vi "appendXMLDetectParam.vi"(8 "Detection Parameters":T1, 9 "error in (no error)":errorcluster, 10 "Parent Device Node":refnum<k20>, 11 "DOM document in":refnum<k20>) -> (0 "error out":errorcluster)   [LabVIEW 2013]
uses:
  <resource>/objmgr/DOMUserDefRef.rc
panel:
  out "R%":sgl
  out "Ry":i32
  out "Rx":i32
  out "Max Intensity%":u8
  out "Max Intensity":i32
  out "Treshold":u8
  out "Contrast":i32
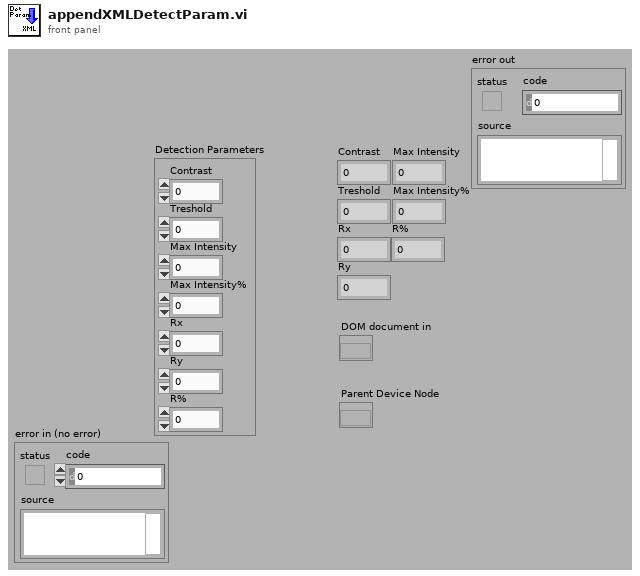
[diagram p1: front panel]
types:
  T1 = cluster{"Contrast":i32, "Treshold":u8, "Max Intensity":i32, "Max Intensity%":u8, "Rx":i32, "Ry":i32, "R%":sgl}
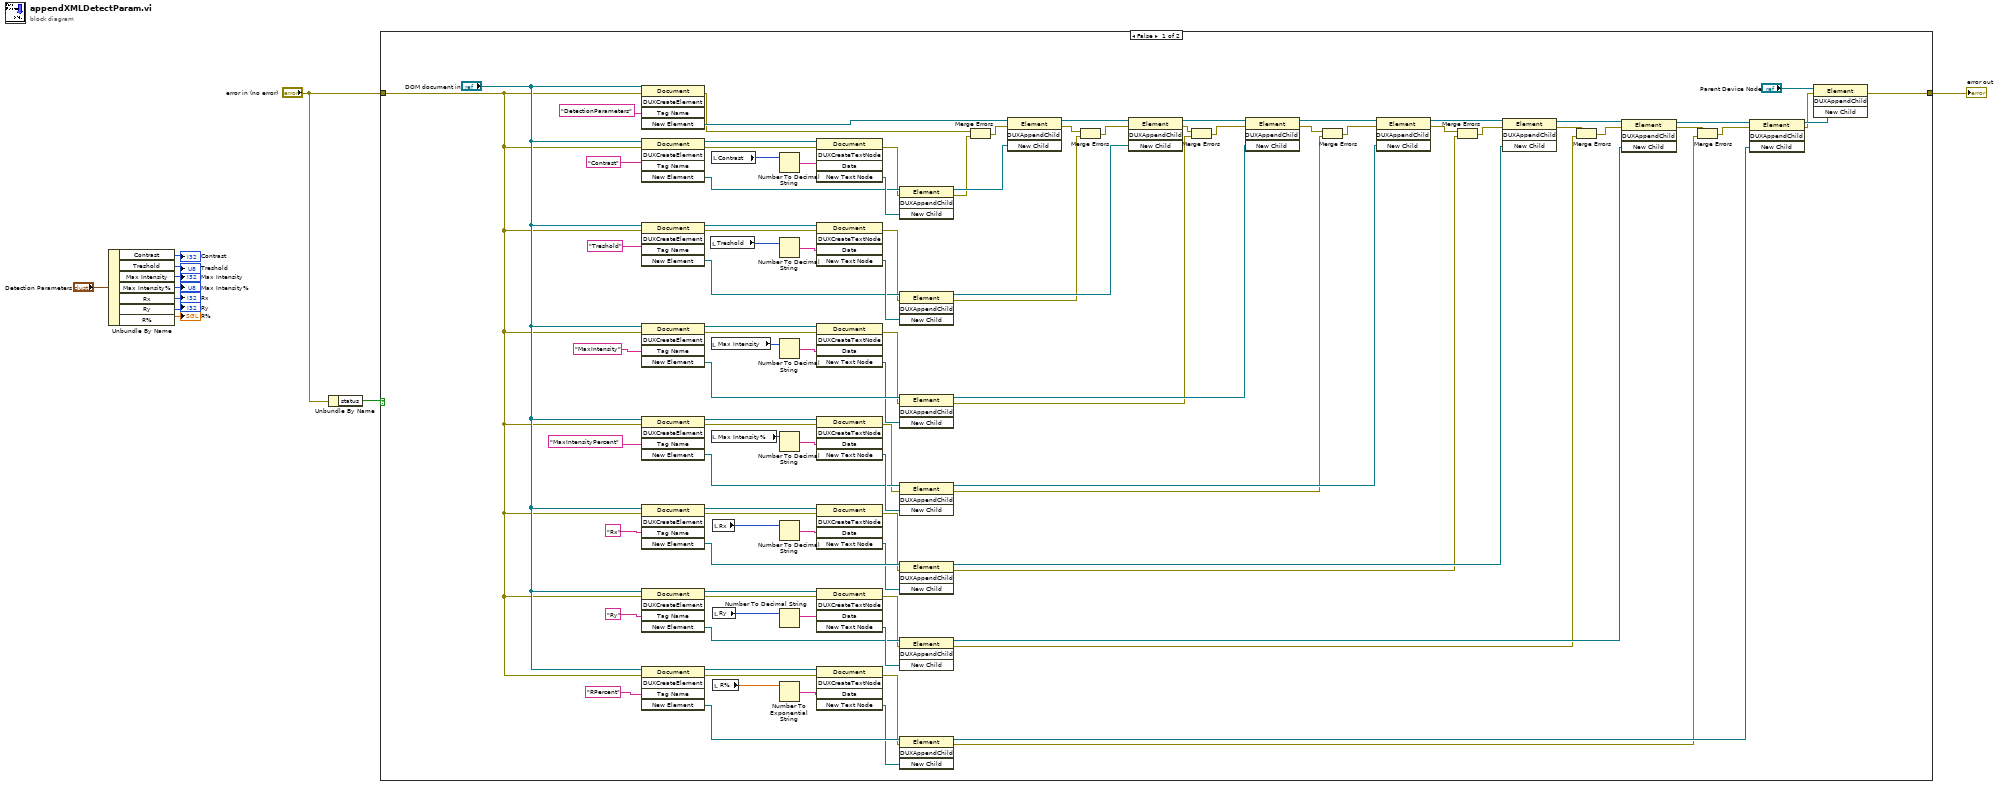
[diagram p0: block diagram]
diagram:
  n1 = Unbundle By Name("Detection Parameters") -> ("Contrast"=→"Contrast":i32, "Treshold"=→"Treshold":u8, "Max Intensity"=→"Max Intensity":i32, "Max Intensity%"=→"Max Intensity%":u8, "Rx"=→"Rx":i32, "Ry"=→"Ry":i32, "R%"=→"R%":sgl)
  n2 = Unbundle By Name("error in (no error)") -> ("status"=w1:bool)
  n3 = case shown="False" w1 {
    tunnel: "error in (no error)" -> [w49 w110]
    tunnel: [w12 w110] -> w3
    frame False {
      n4 = invoke class="Document" method="DUXCreateElement"(reference="DOM document in", error in=w49, "Tag Name"="DetectionParameters") -> (error out=w33:errorcluster, "New Element"=w104:refnum<k20>)  [unwired: 2 in, 3 out]
      n5 = invoke class="Document" method="DUXCreateElement"(reference="DOM document in", error in=w49, "Tag Name"="Contrast") -> (reference out=w103:refnum<k20>, error out=w46:errorcluster, "New Element"=w99:refnum<k20>)  [unwired: 2 in, 2 out]
      n6 = invoke class="Document" method="DUXCreateElement"(reference="DOM document in", error in=w49, "Tag Name"="Treshold") -> (reference out=w106:refnum<k20>, error out=w43:errorcluster, "New Element"=w101:refnum<k20>)  [unwired: 2 in, 2 out]
      n7 = invoke class="Document" method="DUXCreateElement"(reference="DOM document in", error in=w49, "Tag Name"="MaxIntensity") -> (reference out=w93:refnum<k20>, error out=w42:errorcluster, "New Element"=w95:refnum<k20>)  [unwired: 2 in, 2 out]
      n8 = invoke class="Document" method="DUXCreateElement"(reference="DOM document in", error in=w49, "Tag Name"="MaxIntensityPercent") -> (reference out=w90:refnum<k20>, error out=w41:errorcluster, "New Element"=w88:refnum<k20>)  [unwired: 2 in, 2 out]
      n9 = invoke class="Document" method="DUXCreateElement"(reference="DOM document in", error in=w49, "Tag Name"="Rx") -> (reference out=w85:refnum<k20>, error out=w40:errorcluster, "New Element"=w87:refnum<k20>)  [unwired: 2 in, 2 out]
      n10 = invoke class="Document" method="DUXCreateElement"(reference="DOM document in", error in=w49, "Tag Name"="Ry") -> (reference out=w82:refnum<k20>, error out=w47:errorcluster, "New Element"=w80:refnum<k20>)  [unwired: 2 in, 2 out]
      n11 = invoke class="Document" method="DUXCreateElement"(reference="DOM document in", error in=w49, "Tag Name"="RPercent") -> (reference out=w77:refnum<k20>, error out=w48:errorcluster, "New Element"=w79:refnum<k20>)  [unwired: 2 in, 2 out]
      n12 = local read "Treshold"() -> (w65:u8)
      n13 = local read "Max Intensity"() -> (w67:i32)
      n14 = local read "Max Intensity%"() -> (w69:u8)
      n15 = local read "Contrast"() -> (w63:i32)
      n16 = local read "Rx"() -> (w71:i32)
      n17 = local read "Ry"() -> (w73:i32)
      n18 = local read "R%"() -> (w75:sgl)
      n19 = Number To Decimal String(number=w63) -> (decimal integer string=w62:string)  [unwired: 1 in]
      n20 = Number To Decimal String(number=w65) -> (decimal integer string=w64:string)  [unwired: 1 in]
      n21 = Number To Decimal String(number=w67) -> (decimal integer string=w66:string)  [unwired: 1 in]
      n22 = Number To Decimal String(number=w69) -> (decimal integer string=w68:string)  [unwired: 1 in]
      n23 = Number To Decimal String(number=w71) -> (decimal integer string=w70:string)  [unwired: 1 in]
      n24 = Number To Decimal String(number=w73) -> (decimal integer string=w72:string)  [unwired: 1 in]
      n25 = Number To Exponential String(number=w75) -> (E-format string=w74:string)  [unwired: 3 in]
      n26 = invoke class="Document" method="DUXCreateTextNode"(reference=w103, error in=w46, "Data"=w62) -> (error out=w45:errorcluster, "New Text Node"=w100:refnum<k20>)  [unwired: 2 in, 3 out]
      n27 = invoke class="Document" method="DUXCreateTextNode"(reference=w106, error in=w43, "Data"=w64) -> (error out=w44:errorcluster, "New Text Node"=w102:refnum<k20>)  [unwired: 2 in, 3 out]
      n28 = invoke class="Document" method="DUXCreateTextNode"(reference=w93, error in=w42, "Data"=w66) -> (error out=w39:errorcluster, "New Text Node"=w94:refnum<k20>)  [unwired: 2 in, 3 out]
      n29 = invoke class="Document" method="DUXCreateTextNode"(reference=w90, error in=w41, "Data"=w68) -> (error out=w38:errorcluster, "New Text Node"=w89:refnum<k20>)  [unwired: 2 in, 3 out]
      n30 = invoke class="Document" method="DUXCreateTextNode"(reference=w85, error in=w40, "Data"=w70) -> (error out=w37:errorcluster, "New Text Node"=w86:refnum<k20>)  [unwired: 2 in, 3 out]
      n31 = invoke class="Document" method="DUXCreateTextNode"(reference=w82, error in=w47, "Data"=w72) -> (error out=w36:errorcluster, "New Text Node"=w81:refnum<k20>)  [unwired: 2 in, 3 out]
      n32 = invoke class="Document" method="DUXCreateTextNode"(reference=w77, error in=w48, "Data"=w74) -> (error out=w35:errorcluster, "New Text Node"=w78:refnum<k20>)  [unwired: 2 in, 3 out]
      n33 = invoke class="Element" method="DUXAppendChild"(reference=w99, error in=w45, "New Child"=w100) -> (reference out=w98:refnum<k20>, error out=w32:errorcluster)  [unwired: 1 in, 2 out]
      n34 = invoke class="Element" method="DUXAppendChild"(reference=w101, error in=w44, "New Child"=w102) -> (reference out=w97:refnum<k20>, error out=w29:errorcluster)  [unwired: 1 in, 2 out]
      n35 = invoke class="Element" method="DUXAppendChild"(reference=w95, error in=w39, "New Child"=w94) -> (reference out=w55:refnum<k20>, error out=w26:errorcluster)  [unwired: 1 in, 2 out]
      n36 = invoke class="Element" method="DUXAppendChild"(reference=w88, error in=w38, "New Child"=w89) -> (reference out=w54:refnum<k20>, error out=w22:errorcluster)  [unwired: 1 in, 2 out]
      n37 = invoke class="Element" method="DUXAppendChild"(reference=w87, error in=w37, "New Child"=w86) -> (reference out=w53:refnum<k20>, error out=w19:errorcluster)  [unwired: 1 in, 2 out]
      n38 = invoke class="Element" method="DUXAppendChild"(reference=w80, error in=w36, "New Child"=w81) -> (reference out=w52:refnum<k20>, error out=w16:errorcluster)  [unwired: 1 in, 2 out]
      n39 = invoke class="Element" method="DUXAppendChild"(reference=w79, error in=w35, "New Child"=w78) -> (reference out=w51:refnum<k20>, error out=w13:errorcluster)  [unwired: 1 in, 2 out]
      n40 = Merge Errors(w33, w32) -> (w31:errorcluster)
      n41 = invoke class="Element" method="DUXAppendChild"(reference=w104, error in=w31, "New Child"=w98) -> (reference out=w105:refnum<k20>, error out=w30:errorcluster)  [unwired: 1 in, 2 out]
      n42 = Merge Errors(w30, w29) -> (w28:errorcluster)
      n43 = invoke class="Element" method="DUXAppendChild"(reference=w105, error in=w28, "New Child"=w97) -> (reference out=w61:refnum<k20>, error out=w27:errorcluster)  [unwired: 1 in, 2 out]
      n44 = Merge Errors(w27, w26) -> (w25:errorcluster)
      n45 = invoke class="Element" method="DUXAppendChild"(reference=w61, error in=w25, "New Child"=w55) -> (reference out=w60:refnum<k20>, error out=w23:errorcluster)  [unwired: 1 in, 2 out]
      n46 = Merge Errors(w23, w22) -> (w24:errorcluster)
      n47 = invoke class="Element" method="DUXAppendChild"(reference=w60, error in=w24, "New Child"=w54) -> (reference out=w59:refnum<k20>, error out=w20:errorcluster)  [unwired: 1 in, 2 out]
      n48 = Merge Errors(w20, w19) -> (w21:errorcluster)
      n49 = invoke class="Element" method="DUXAppendChild"(reference=w59, error in=w21, "New Child"=w53) -> (reference out=w58:refnum<k20>, error out=w18:errorcluster)  [unwired: 1 in, 2 out]
      n50 = Merge Errors(w18, w16) -> (w17:errorcluster)
      n51 = invoke class="Element" method="DUXAppendChild"(reference=w58, error in=w17, "New Child"=w52) -> (reference out=w57:refnum<k20>, error out=w15:errorcluster)  [unwired: 1 in, 2 out]
      n52 = Merge Errors(w15, w13) -> (w14:errorcluster)
      n53 = invoke class="Element" method="DUXAppendChild"(reference=w57, error in=w14, "New Child"=w51) -> (reference out=w56:refnum<k20>, error out=w34:errorcluster)  [unwired: 1 in, 2 out]
      n54 = invoke class="Element" method="DUXAppendChild"(reference="Parent Device Node", error in=w34, "New Child"=w56) -> (error out=w12:errorcluster)  [unwired: 1 in, 3 out]
    }
    frame True {
    }
  }
  "error out" <- w3
